vi "launcher.vi"() -> ()   [LabVIEW 2023]
uses:
  SLM_Controller/SLM_Controller/SLM_Controller.lvclass
  C:/Program Files/National Instruments/LabVIEW 2023/vi.lib/ActorFramework/Actor/Actor.lvclass
  Top_Controllers/Cam_SLM_Controller/Cam_SLM_Controller.lvclass
  Camera_Controller/Camera_Controller/Camera_Controller.lvclass
  <vilib>/ActorFramework/Actor/Actor.lvclass
panel:
  in  "Stop":bool
  in  "SLM+Cam":bool
  in  "Camera":bool
  in  "SLM":bool
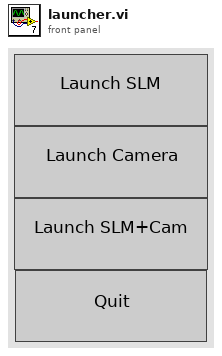
[diagram p1: front panel]
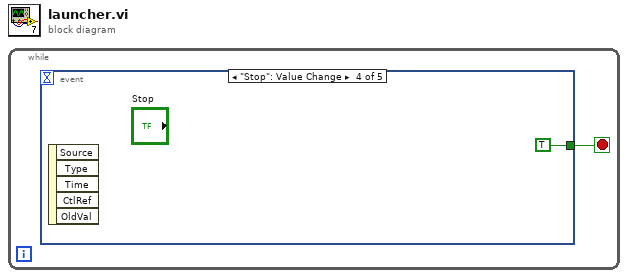
[diagram p0: block diagram]
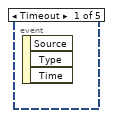
[diagram p2: hidden frame]
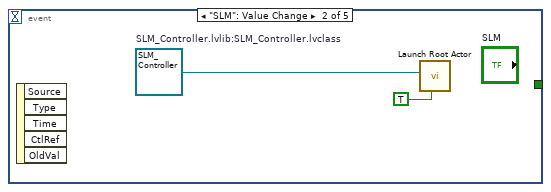
[diagram p3: hidden frame]
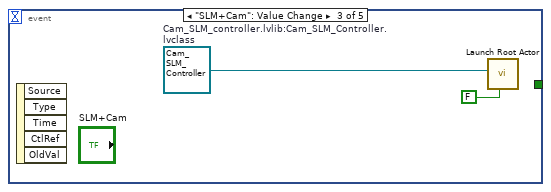
[diagram p4: hidden frame]
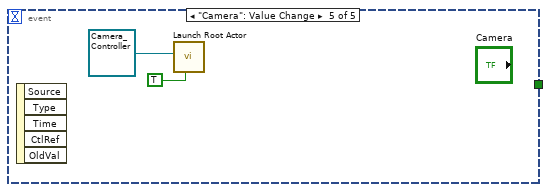
[diagram p5: hidden frame]
diagram:
  n1 = while {
    stop <- w1 stop-if-true
    n2 = event shown="[3] \"Stop\": Value Change" {
      selector: _ -> [_ _ _ _ _]
      dyn-events: _ -> [_ _ _ _ _]
      timeout: _ -> [_ _ _ _ _]
      tunnel: [_ _ _ TRUE _] -> w1
      event Timeout {
        n3 = event-data() -> ()  [unwired: 1 in, 3 out]
      }
      event "SLM": Value Change {
        w2 = refnum<class "SLM_Controller.lvclass"> refnum  # SLM_Controller.lvlib:SLM_Controller.lvclass
        n4 = event-data() -> ()  [unwired: 1 in, 5 out]
        n5 = call <vilib>:"Launch Root Actor.vi"("Open Actor Core front panel? (F)"=TRUE, "Actor"=w2) -> ()  [unwired: 8 in, 2 out]
      }
      event "SLM+Cam": Value Change {
        w4 = refnum<class "Cam_SLM_Controller.lvclass"> refnum  # Cam_SLM_controller.lvlib:Cam_SLM_Controller.lvclass
        n6 = event-data() -> ()  [unwired: 1 in, 5 out]
        n7 = call <vilib>:"Launch Root Actor.vi"("Open Actor Core front panel? (F)"=FALSE, "Actor"=w4) -> ()  [unwired: 8 in, 2 out]
      }
      event "Stop": Value Change {
        n8 = event-data() -> ()  [unwired: 1 in, 5 out]
      }
      event "Camera": Value Change {
        n9 = event-data() -> ()  [unwired: 1 in, 5 out]
        n10 = call <vilib>:"Launch Root Actor.vi"("Open Actor Core front panel? (F)"=TRUE, "Actor"=refnum<class "Camera_Controller.lvclass"> refnum ("Camera_Controller.lvlib:Camera_Controller.lvclass")) -> ()  [unwired: 8 in, 2 out]
      }
    }
  }
